vi "DataCollect.vi"() -> ()   [LabVIEW 2009]
uses:
  BaudRateSelector.ctl
  GlobalVariables.vi
  <vilib>/Platform/TimedLoop/XDataNode/XDataNode.xnode
  <vilib>/Platform/TimedLoop/XDataNode/loadlvalarms.vi
  <vilib>/Platform/TimedLoop/XDataNode/timing_clust.ctl
  <vilib>/Platform/TimedLoop/XDataNode/nitl_modes.ctl
  <vilib>/Platform/TimedLoop/XDataNode/wakeup.ctl
  <vilib>/Utility/file.llb/Write To Spreadsheet File (I64).vi
  <vilib>/Utility/file.llb/Write To Spreadsheet File (DBL).vi
  <vilib>/Utility/file.llb/Write To Spreadsheet File (string).vi
  <vilib>/Platform/TimedLoop/XDataNode/XDNodeRunTimeDep.lvlib
panel:
  in  "Reset Trial #":bool
  in  "Position Trial":bool
  in  "Trial #":i32=1 min=1 step=1
  in  "Experiment #":i32 min=0 step=1
  out "RH Cal Warning":bool
  in  "RH Calibration":string="RH_Calibration1.cal"
  out "LH Cal Warning":bool
  in  "LH Calibration":string="LH_Calibration1.cal"
  in  "Subject Initials":string="Default"
  in  "Start/Mark":bool
  out "RH Raw":u8[](array[numeric])
  out "RH Degrees":dbl[](array[numeric]) format="%7.2f"
  out "Sensor Names":string[](array[string])
  out "LH Degrees":dbl[](array[numeric]) format="%7.2f"
  out "LH Raw":u8[](array[numeric])
  out "RH Movement":dbl(graph)
  in  "RH Glove":bool=TRUE
  in  "LH Glove":bool=TRUE
  in  "Polhemus":bool=TRUE
  out "LH Movement":dbl(graph)
  out "Time":dbl
  out "Hand Position Graph":cluster{sgl, sgl}[](graph)
  in  "stop":bool
  in  "RH COM Port":refnum<visa-resource-name>="COM2"
  in  "LH COM Port":refnum<visa-resource-name>="COM1"
  out "Titles":string[](array[string])
  out "Interpreted Values":sgl[](array[numeric]) format="%.2f"
  in  "Parity":enum16{"None", "Odd", "Even", "Mark", "Space"}(ring)
  in  "Data Bits":u16=8 min=7 max=8 step=1
  in  "Baud Rate":T1=115200 items=["1200"=1200, "2400"=2400, "4800"=4800, "9600"=9600, "19200"=19200, "38400"=38400, "57600"=57600, "115200"=115200]
  in  "Polhemus COM Port":refnum<visa-resource-name>="COM3"
  # "(Pg Down)"
  # "(Pg Up)"
  # "Collect Data From:"
  # "If Data Bits = 8, Parity must be \"None\""
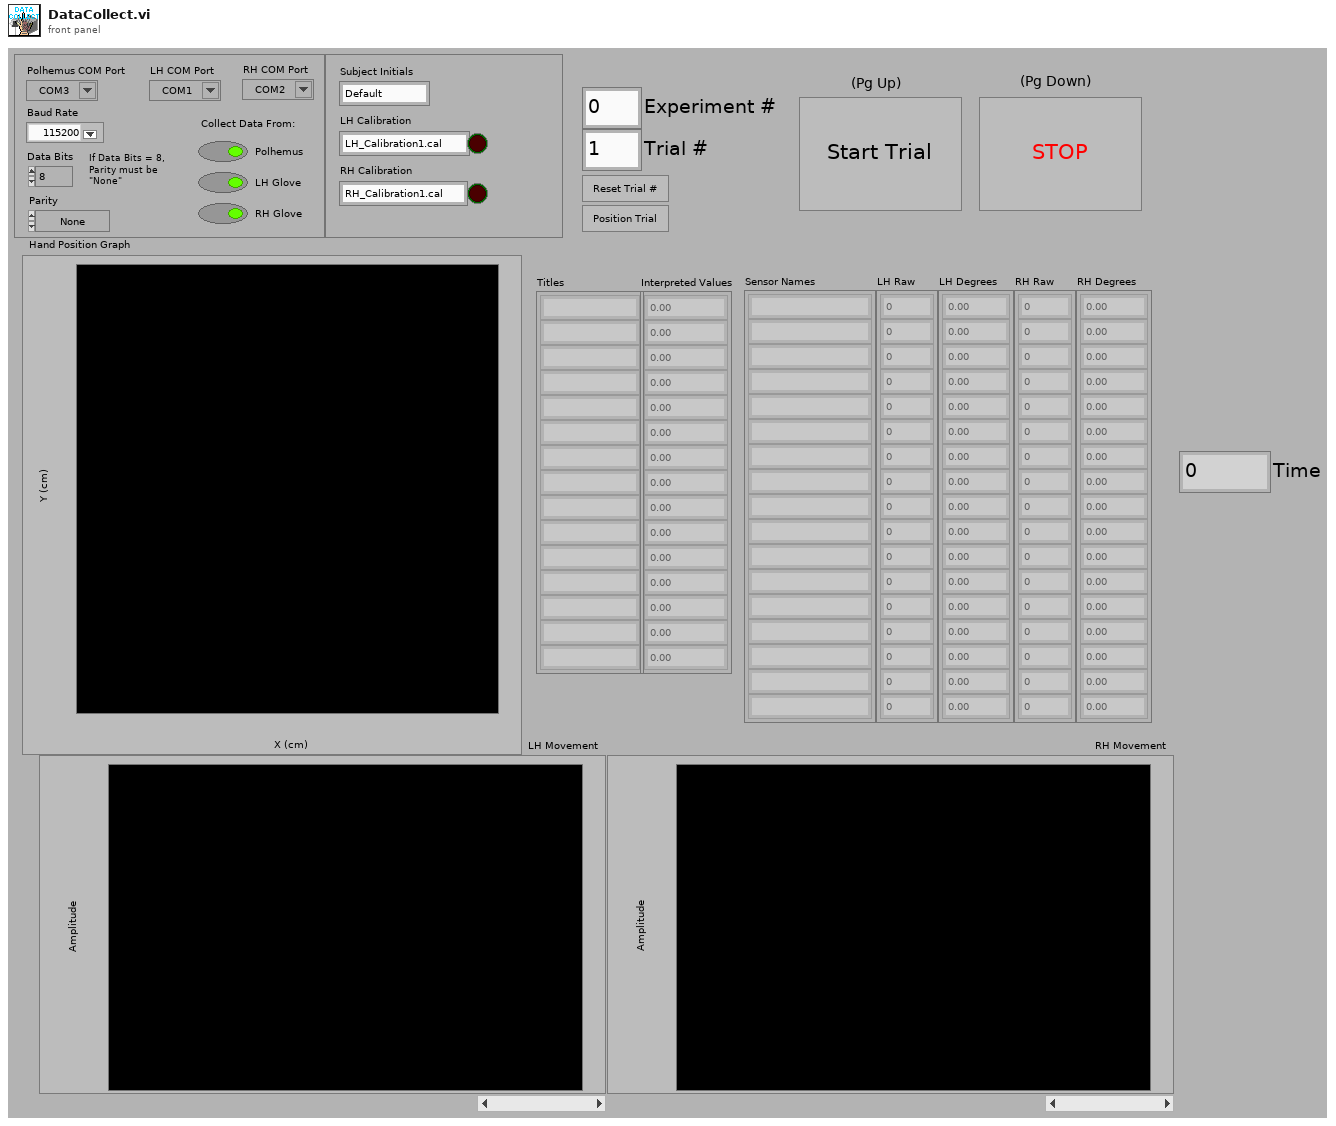
[diagram p1: front panel]
types:
  T1 = typedef "BaudRateSelector.ctl" = u32
  T2 = enum8{"Enabled", "Disabled", "Disabled and Grayed Out"}
  T3 = cluster{"#Bytes":i32[], "Titles":string[], "Format":enum16{"ASCII", "Binary"}, "Units":enum16{"Inches", "Centimeters"}, "Station State":bool[], "#Line Feeds":i32}
  T4 = typedef "XDNodeRunTimeDep.lvlib/timing_clust.ctl" = cluster{"Expected End [f-1]":u64, "Actual End [f-1]":u64, "Finished Late? [f-1]":bool, "Expected End [i-1]":u64, "Actual End [i-1]":u64, "Finished Late? [i-1]":bool, "Expected Start [i]":u64, "Actual Start [i]":u64, "Expected Start [f]":u64, "Actual Start [f]":u64, "Source Name":string, "Structure Name":string, "Period":i64, "Deadline":i64, "Offset":i64, "Start":i64, "Priority":i32, "Timeout":i32, "Mode":T5, "Wakeup Reason":T6, "Error":errorcluster, "Source Type":string, "Secondary Source Type":string, "Global End Time":u64, "Global Start Time":u64, "Frame Duration":u64, "Iteration Duration":u64, "Assigned CPU":i32, "I/O Scan Engine Mode":u32}
  T5 = typedef "XDNodeRunTimeDep.lvlib/nitl_modes.ctl" = enum32{"No Change", "Process missed periods, maintain original phase", "Discard missed periods, maintain original phase", "Process missed periods, ignore original phase", "Discard missed periods, ignore original phase"}
  T6 = typedef "XDNodeRunTimeDep.lvlib/wakeup.ctl" = enum32{"Normal", "Aborted", "Asynchronous wakeup", "Timing source error", "Timed loop error", "Timeout"}
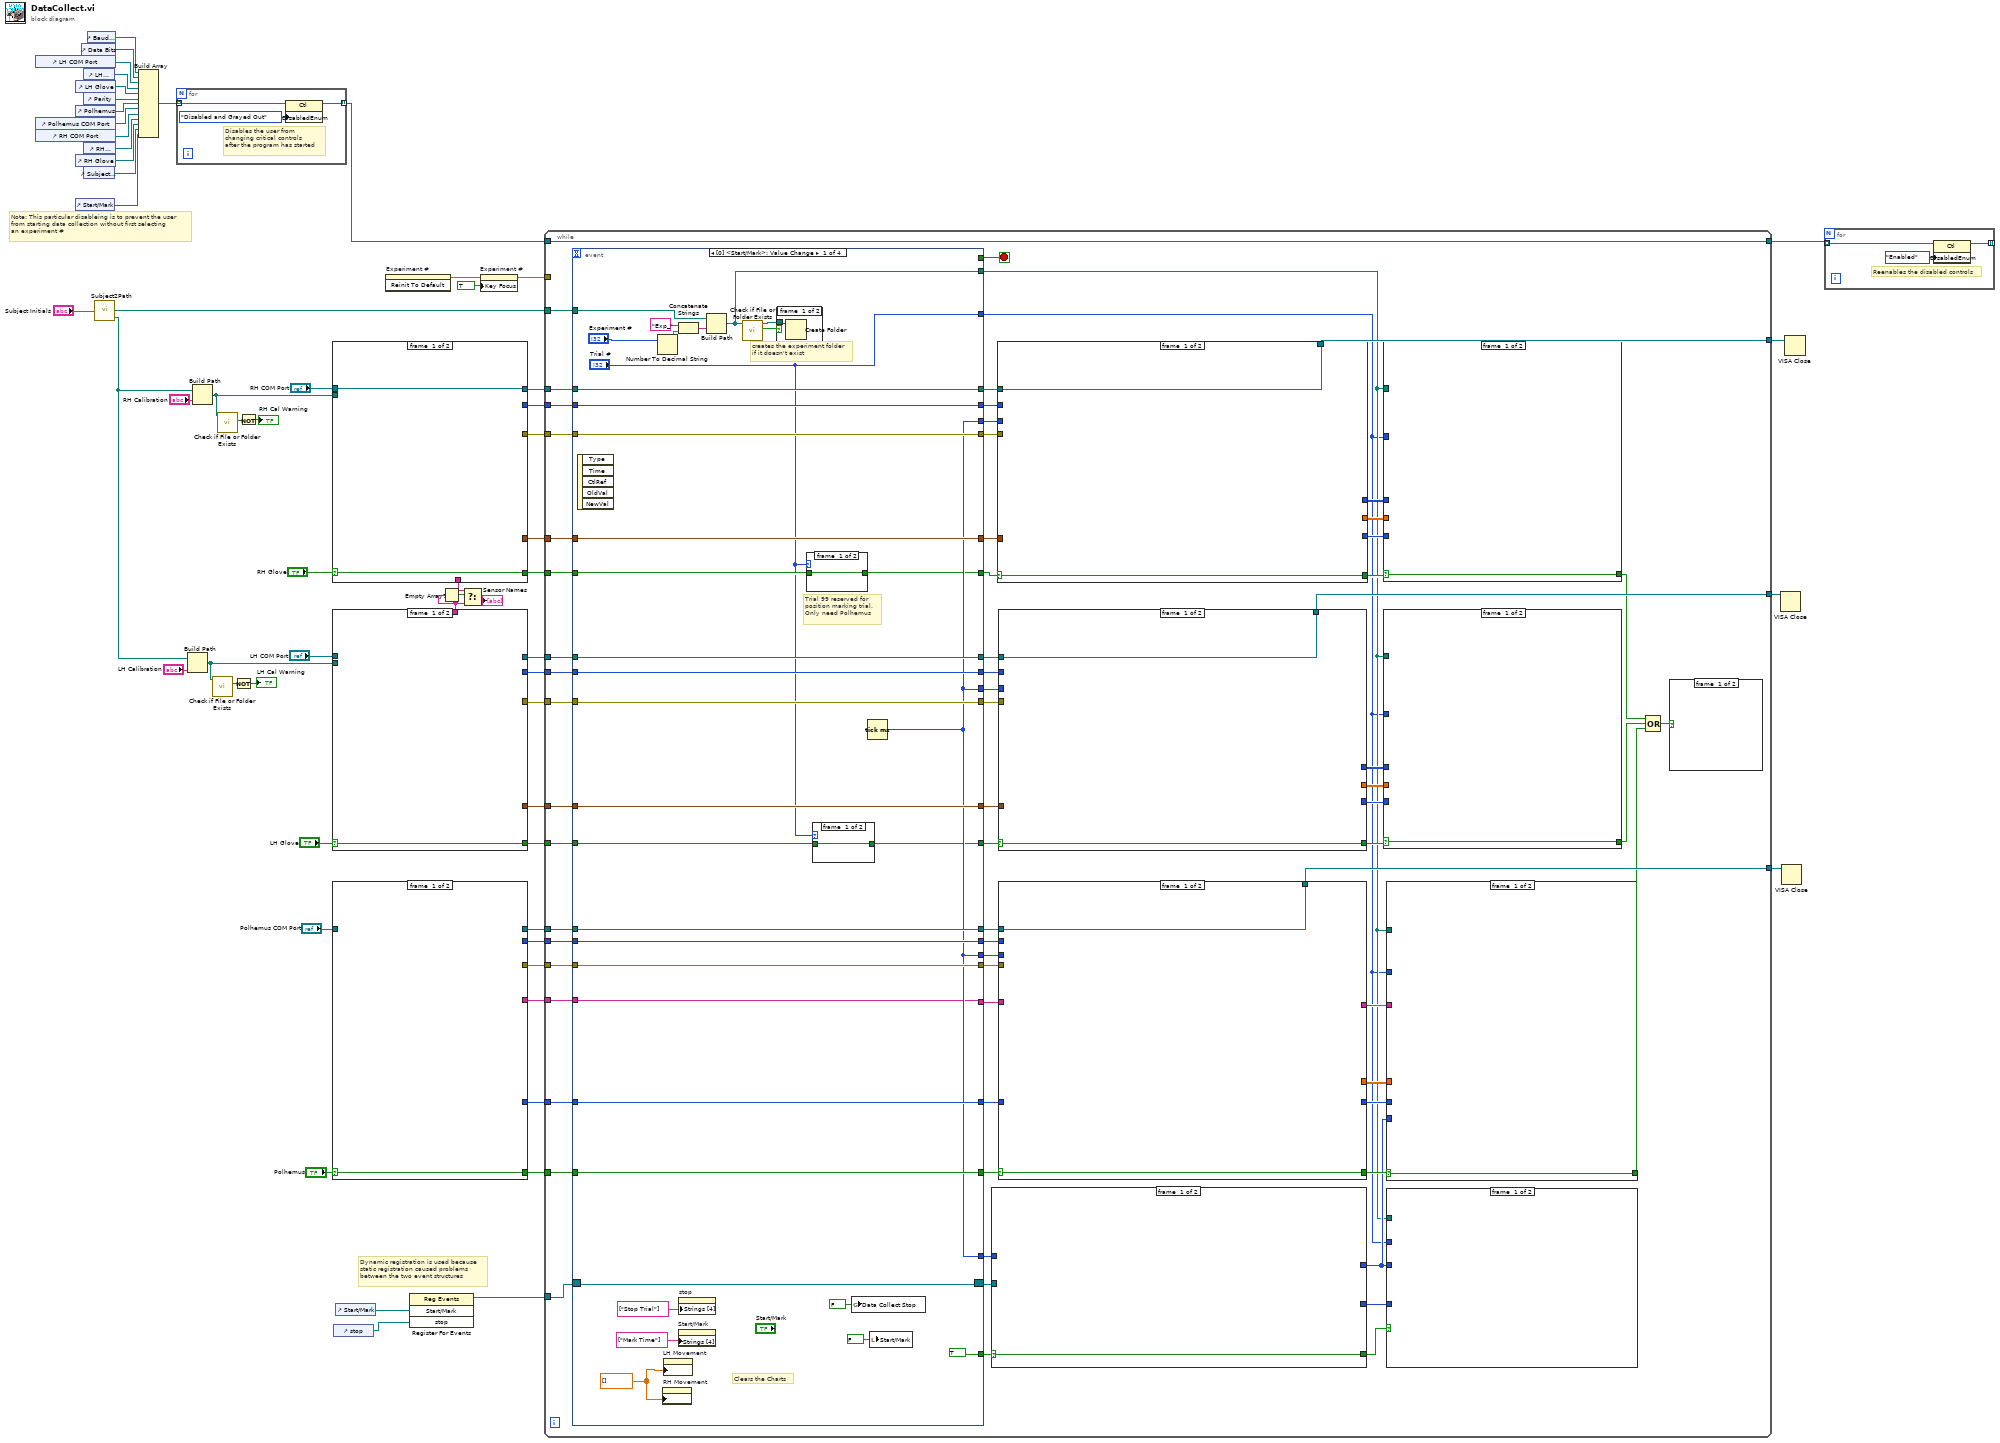
[diagram p0: block diagram]
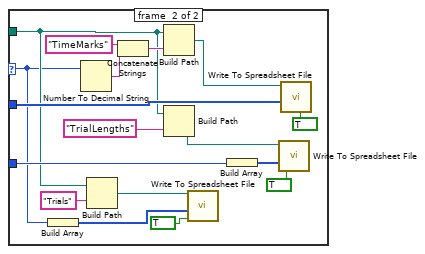
[diagram p3: hidden frame]
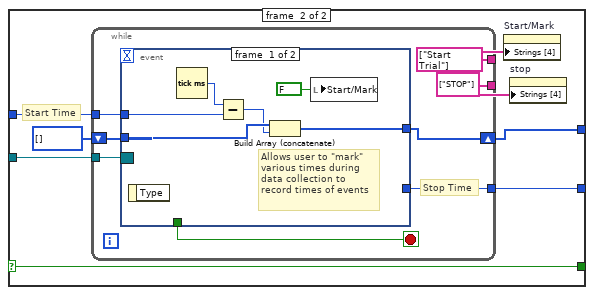
[diagram p4: hidden frame]
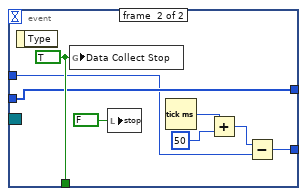
[diagram p5: hidden frame]
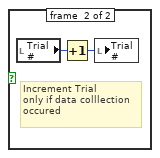
[diagram p6: hidden frame]
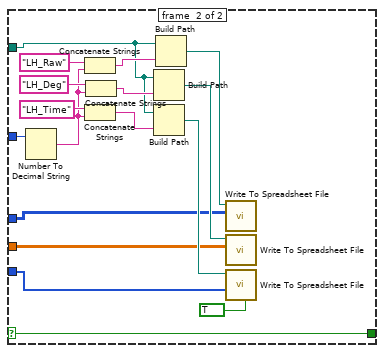
[diagram p7: hidden frame]
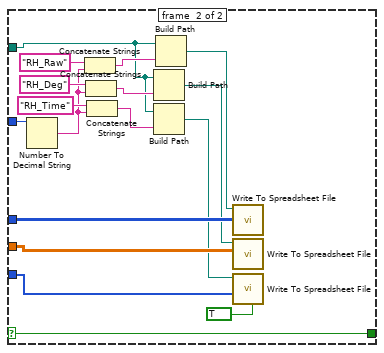
[diagram p8: hidden frame]
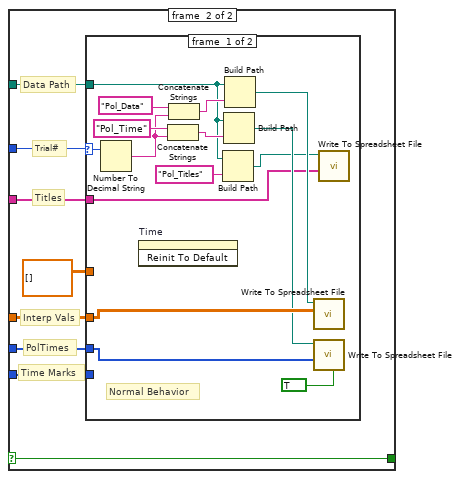
[diagram p9: hidden frame]
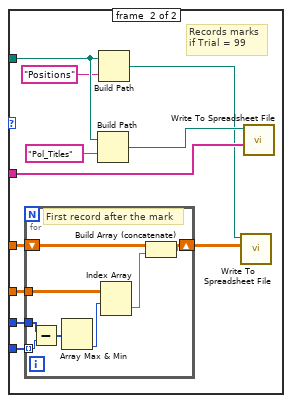
[diagram p10: hidden frame]
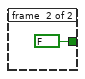
[diagram p11: hidden frame]
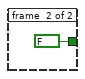
[diagram p12: hidden frame]
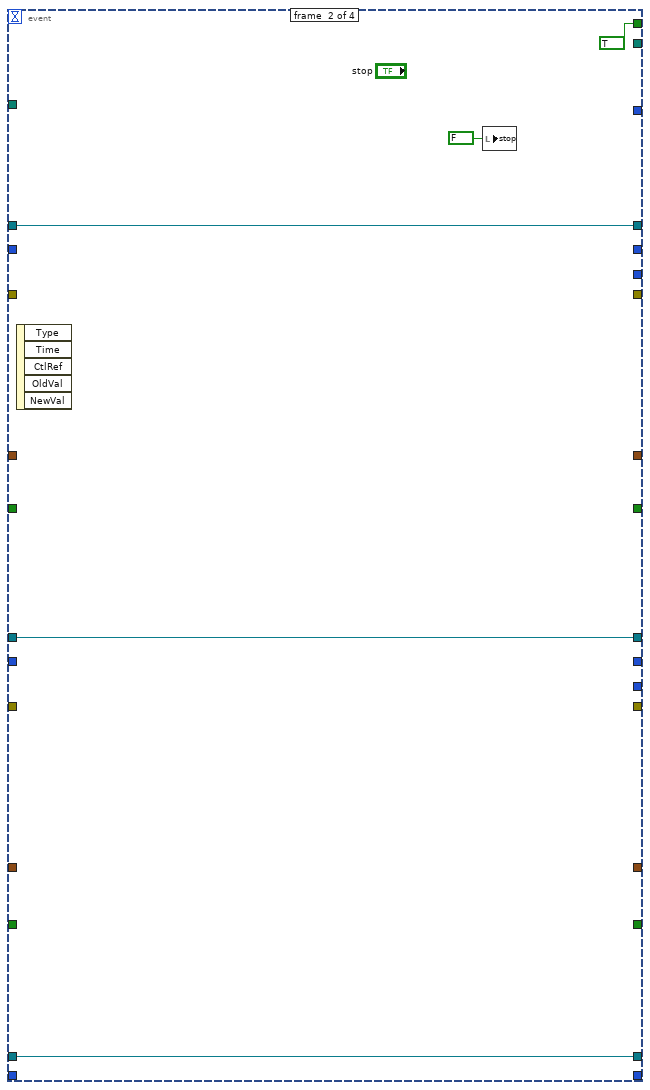
[diagram p14: hidden frame]
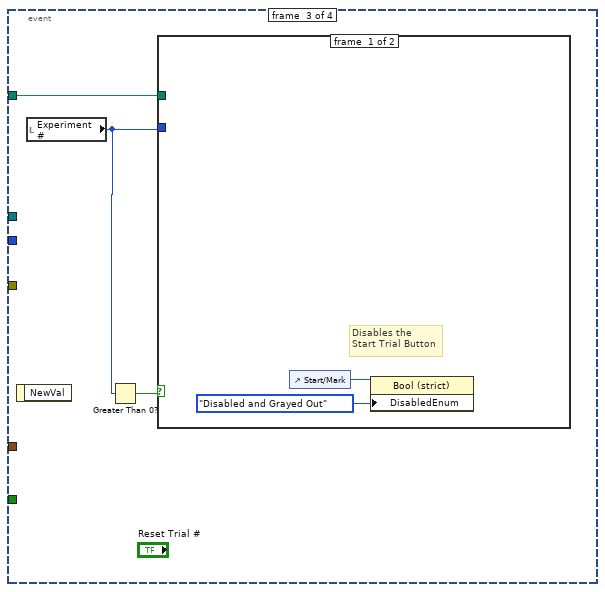
[diagram p15: hidden frame]
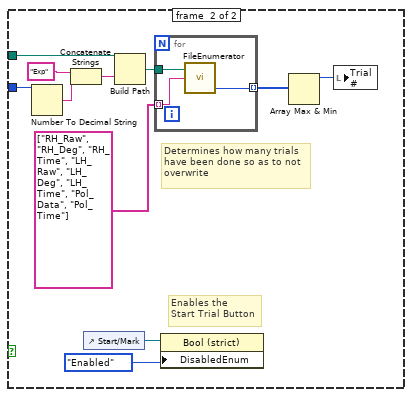
[diagram p16: hidden frame]
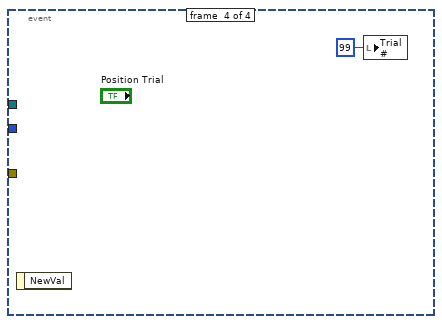
[diagram p17: hidden frame]
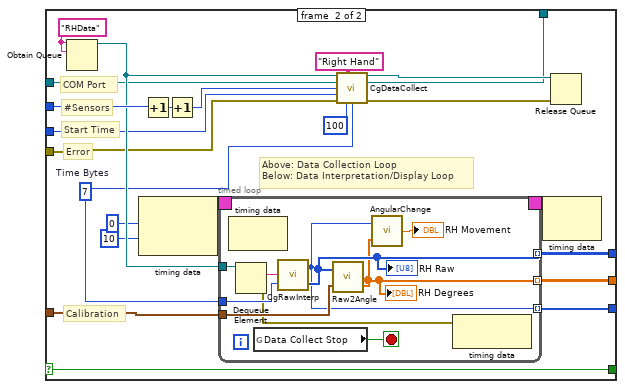
[diagram p18: hidden frame]
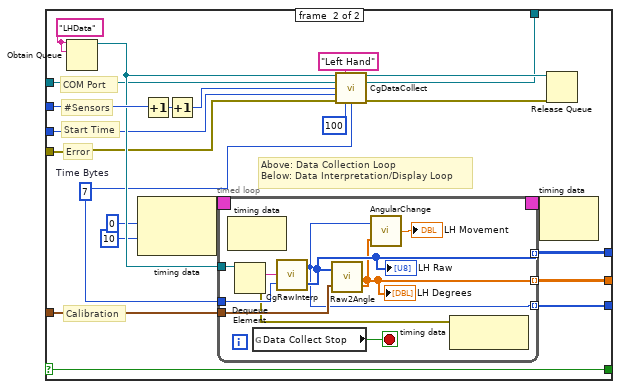
[diagram p19: hidden frame]
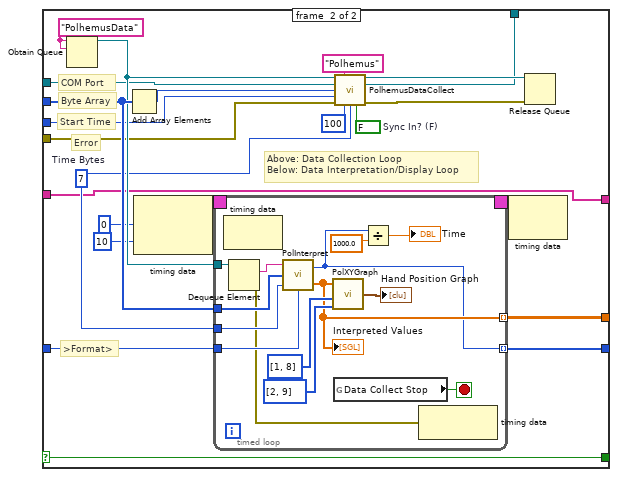
[diagram p20: hidden frame]
diagram:
  # "Dynamic registration is used because\nstatic registration caused problems\nbetween the two event structures"
  # "Note: This particular disableing is to prevent the user\nfrom starting data collection without first selecting\nan experiment #"
  n1 = control-ref of="LH COM Port"() -> (w36:refnum<vi>)
  n2 = control-ref of="Polhemus COM Port"() -> (w31:refnum<vi>)
  n3 = control-ref of="RH COM Port"() -> (w30:refnum<vi>)
  n4 = control-ref of="Start/Mark"() -> (w11:refnum<vi>)
  n5 = control-ref of="LH Glove"() -> (w34:refnum<vi>)
  n6 = control-ref of="Polhemus"() -> (w32:refnum<vi>)
  n7 = control-ref of="RH Glove"() -> (w28:refnum<vi>)
  n8 = control-ref of="Data Bits"() -> (w37:refnum<vi>)
  n9 = control-ref of="LH Calibration"() -> (w35:refnum<vi>)
  n10 = control-ref of="Subject Initials"() -> (w27:refnum<vi>)
  n11 = control-ref of="Parity"() -> (w33:refnum<vi>)
  n12 = control-ref of="RH Calibration"() -> (w29:refnum<vi>)
  n13 = control-ref of="Baud Rate"() -> (w26:refnum<vi>)
  n14 = call "Subject2Path.vi"("Subject Initials"="Subject Initials") -> ("Data Path"=w23:path, "Calibration Path"=w14:path)  [unwired: 1 in, 1 out]
  n15 = Build Array(w26, w37, w36, w35, w34, w33, w32, w31, w30, w29, w28, w27, w11) -> (w25:refnum<vi>[])
  n16 = for {
    tunnel: w25 -> [w65] mode=indexing
    tunnel: [w63] -> w13 mode=indexing
    # "Disables the user from\nchanging critical controls\nafter the program has started"
    n17 = property class="Ctl"(reference=w65, "DisabledEnum"=T2."Disabled and Grayed Out" ("Disabled")) -> (reference out=w63:refnum<vi>)  [unwired: 1 in, 1 out]
  }
  n18 = Build Path(base path=w14, name or relative path="LH Calibration") -> (appended path=w17:path)
  n19 = Build Path(base path=w14, name or relative path="RH Calibration") -> (appended path=w21:path)
  n20 = call <vilib>:"Check if File or Folder Exists.vi"("path"=w17) -> ("file or folder exists?"=w16:bool)  [unwired: 8 in, 2 out]
  n21 = call <vilib>:"Check if File or Folder Exists.vi"("path"=w21) -> ("file or folder exists?"=w20:bool)  [unwired: 8 in, 2 out]
  n22 = Not(x=w16) -> (.not. x?=→"LH Cal Warning":bool)
  n23 = Not(x=w20) -> (.not. x?=→"RH Cal Warning":bool)
  n24 = case shown="True" "RH Glove" {
    selector: "RH Glove" -> [w67 w69]
    tunnel: [w66 w75] -> w47
    tunnel: [_ w74] -> w46
    tunnel: [_ w73] -> w45
    tunnel: [_ w72] -> w44
    tunnel: [_ w71] -> w56
    tunnel: [w67 w69] -> w43
    tunnel: "RH COM Port" -> [w66 w70]
    tunnel: w21 -> [_ w68]
    frame #0 {
    }
    frame #1 {
      # "Initializes the RH Glove"
      n25 = call "CgInit.vi"("Calibration File"=w68, "VISA resource name"=w70) -> ("error out"=w73:errorcluster, "Sensor Names"=w71:string[], "#Sensors"=w74:i32, "VISA resource name out"=w75:refnum<visa-resource-name>, "Calibration Array"=w72:cluster{"Offset":dbl, "Gain":dbl}[])  [unwired: 3 in]
    }
  }
  n26 = case shown="True" "LH Glove" {
    selector: "LH Glove" -> [w76 w78]
    tunnel: [_ w84] -> w62
    tunnel: [_ w83] -> w41
    tunnel: [_ w82] -> w61
    tunnel: [_ w81] -> w40
    tunnel: [_ w80] -> w53
    tunnel: [w76 w78] -> w51
    tunnel: "LH COM Port" -> [_ w79]
    tunnel: w17 -> [_ w77]
    frame #0 {
    }
    frame #1 {
      # "Initializes the LH Glove"
      n27 = call "CgInit.vi"("Calibration File"=w77, "VISA resource name"=w79) -> ("error out"=w81:errorcluster, "Sensor Names"=w80:string[], "#Sensors"=w84:i32, "VISA resource name out"=w83:refnum<visa-resource-name>, "Calibration Array"=w82:cluster{"Offset":dbl, "Gain":dbl}[])  [unwired: 3 in]
    }
  }
  n28 = case shown="True" "Polhemus" {
    selector: "Polhemus" -> [w85 w88]
    tunnel: [_ w96] -> w60
    tunnel: [_ w95] -> w59
    tunnel: [_ w94] -> w58
    tunnel: [_ w93] -> w57
    tunnel: [w85 w88] -> w52
    tunnel: "Polhemus COM Port" -> [_ w87]
    tunnel: [_ w86] -> w7
    frame #0 {
    }
    frame #1 {
      # "Initializes the Polhemus"
      n29 = call "PolInit.vi"("VISA resource name"=w87, "Baud Rate"="Baud Rate", "Data Bits"="Data Bits", "Parity"="Parity") -> ("VISA resource name out"=w94:refnum<visa-resource-name>, "Polhemus Info"=w89:T3, "error out"=w93:errorcluster)  [unwired: 9 in]
      n30 = Unbundle By Name(w89) -> ("#Bytes"=w96:i32[], "Titles"=w86:string[], "Format"=w95:enum16{"ASCII", "Binary"})  [unwired: 2 out]
      "Titles" <- w86
    }
  }
  n31 = control-ref of="stop"() -> (w4:refnum<vi>)
  n32 = control-ref of="Start/Mark"() -> (w6:refnum<vi>)
  n33 = invoke on="Experiment #" class="DigNum (strict)" method="Reinit To Default"() -> (error out=w3:errorcluster)  [unwired: 3 in, 2 out]
  n34 = register-events(w6, w4) -> (reference out=w5:refnum<event-registration>)  [unwired: 2 in, 1 out]
  n35 = Empty Array?(array=w53) -> (empty?=w55:bool)
  n36 = Select(t=w56, s=w55, f=w53) -> (s? t:f=→"Sensor Names":string[])
  n37 = property on="Experiment #" class="DigNum (strict)"(error in=w3, "Key Focus"=TRUE) -> (error out=w2:errorcluster)  [unwired: 1 in, 1 out]
  n38 = while {
    tunnel: w62 -> [w156]
    tunnel: w61 -> [w154]
    tunnel: w60 -> [w151]
    tunnel: w59 -> [w149]
    tunnel: w58 -> [w152]
    tunnel: w57 -> [w150]
    tunnel: w52 -> [w148]
    tunnel: w51 -> [w153]
    tunnel: w47 -> [w162]
    tunnel: w46 -> [w161]
    tunnel: w45 -> [w160]
    tunnel: w44 -> [w159]
    tunnel: w43 -> [w158]
    tunnel: w41 -> [w157]
    tunnel: w40 -> [w155]
    tunnel: w23 -> [w128]
    tunnel: w13 -> [w127]
    tunnel: [w127] -> w12
    tunnel: [w126] -> w8
    tunnel: [w125] -> w9
    tunnel: [w124] -> w10
    tunnel: w7 -> [w108]
    tunnel: w5 -> [w103]
    tunnel: w2 -> [_]
    stop <- w129 stop-if-true
    n39 = event shown="[0] <Start/Mark>: Value Change" {
      selector: w103 -> [w303 _ _ _]
      dyn-events: [w303 _ _ _] -> w102
      timeout: _ -> [_ _ _ _]
      tunnel: w162 -> [w321 w340 _ _]
      tunnel: w161 -> [w322 _ _ _]
      tunnel: w160 -> [w323 _ _ _]
      tunnel: w159 -> [w324 _ _ _]
      tunnel: w158 -> [w300 _ _ _]
      tunnel: w157 -> [w312 w339 _ _]
      tunnel: w156 -> [w311 _ _ _]
      tunnel: w155 -> [w310 _ _ _]
      tunnel: w154 -> [w325 _ _ _]
      tunnel: w153 -> [w298 _ _ _]
      tunnel: w152 -> [w326 w338 _ _]
      tunnel: w151 -> [w327 _ _ _]
      tunnel: w150 -> [w328 _ _ _]
      tunnel: w149 -> [w329 _ _ _]
      tunnel: w148 -> [w330 _ _ _]
      tunnel: [w330 _ _ _] -> w147
      tunnel: [w329 _ _ _] -> w146
      tunnel: [w328 _ _ _] -> w145
      tunnel: [w327 _ _ _] -> w144
      tunnel: [w326 w338 _ _] -> w143
      tunnel: [w297 _ _ _] -> w142
      tunnel: [w325 _ _ _] -> w141
      tunnel: [w310 _ _ _] -> w140
      tunnel: [w311 _ _ _] -> w139
      tunnel: [w312 w339 _ _] -> w138
      tunnel: [w299 _ _ _] -> w137
      tunnel: [w324 _ _ _] -> w136
      tunnel: [w323 _ _ _] -> w135
      tunnel: [w322 _ _ _] -> w134
      tunnel: [w321 w340 _ _] -> w133
      tunnel: [w309 _ _ _] -> w105
      tunnel: [w309 _ _ _] -> w132
      tunnel: [w309 _ _ _] -> w131
      tunnel: [w309 _ _ _] -> w130
      tunnel: [_ TRUE ("stop") _ _] -> w129
      tunnel: w128 -> [w318 _ w342 _]
      tunnel: [w315 _ _ _] -> w99
      tunnel: ["Trial #" _ _ _] -> w98
      tunnel: [w306 _ _ _] -> w107
      tunnel: w108 -> [w306 _ _ _]
      tunnel: [TRUE _ _ _] -> w101
      event #0 {
        w308 = dbl[] [] ("History Data")
        # "Trial 99 reserved for\nposition marking trial.\nOnly need Polhemus"
        # "Clears the Charts"
        # "creates the experiment folder\nif it doesn't exist"
        n40 = event-data() -> ()  [unwired: 1 in, 5 out]
        n41 = Number To Decimal String(number="Experiment #") -> (decimal integer string=w319:string)  [unwired: 1 in]
        n42 = property on="RH Movement" class="WFChart (strict)"("History Data"=w308) -> ()  [unwired: 2 in, 2 out]
        n43 = property on="LH Movement" class="WFChart (strict)"("History Data"=w308) -> ()  [unwired: 2 in, 2 out]
        n44 = Concatenate Strings("Exp_", w319) -> (w317:string)
        n45 = property on="Start/Mark" class="Bool (strict)"("Strings [4]"=string[] ["Mark Time"]) -> ()  [unwired: 2 in, 2 out]
        n46 = property on="stop" class="Bool (strict)"("Strings [4]"=string[] ["Stop Trial"]) -> ()  [unwired: 2 in, 2 out]
        n47 = Build Path(base path=w318, name or relative path=w317) -> (appended path=w315:path)
        n48 = call <vilib>:"Check if File or Folder Exists.vi"("path"=w315) -> ("file or folder exists?"=w314:bool, "dup path"=w313:path)  [unwired: 8 in, 1 out]
        n49 = case shown="False" w314 {
          tunnel: w313 -> [w335 _]
          frame #0 {
            n50 = Create Folder(path (use dialog)=w335) -> ()  [unwired: 2 in, 3 out]
          }
          frame #1 {
          }
        }
        n51 = case shown="Default" "Trial #" {
          tunnel: w300 -> [w333 _]
          tunnel: [w333 FALSE] -> w299
          frame #0 {
          }
          frame #1 {
          }
        }
        n52 = case shown="Default" "Trial #" {
          tunnel: w298 -> [w331 _]
          tunnel: [w331 FALSE] -> w297
          frame #0 {
          }
          frame #1 {
          }
        }
        n53 = global write "GlobalVariables.vi" "Data Collect Stop"(FALSE ("Data Collect Stop")) -> ()
        n54 = Tick Count (ms)() -> (millisecond timer value=w309:u32)
        n55 = local write "Start/Mark"(FALSE ("Start/Mark")) -> ()
      }
      event #1 {
        n56 = event-data() -> ()  [unwired: 1 in, 5 out]
        n57 = local write "stop"(FALSE ("stop")) -> ()
      }
      event #2 {
        n58 = event-data() -> ()  [unwired: 1 in, 1 out]
        n59 = local read "Experiment #"() -> (w341:i32)
        n60 = Greater Than 0?(x=w341) -> (x > 0?=w343:bool)
        n61 = case shown="True" w343 {
          tunnel: w342 -> [_ w351]
          tunnel: w341 -> [_ w354]
          frame #0 {
            # "Disables the\nStart Trial Button"
            n62 = control-ref of="Start/Mark"() -> (w344:refnum<vi>)
            n63 = property class="Bool (strict)"(reference=w344, "DisabledEnum"=T2."Disabled and Grayed Out" ("Disabled")) -> ()  [unwired: 1 in, 2 out]
          }
          frame #1 {
            # "Determines how many trials have been done so as to not overwrite"
            # "Enables the\nStart Trial Button"
            n64 = Number To Decimal String(number=w354) -> (decimal integer string=w352:string)  [unwired: 1 in]
            n65 = Concatenate Strings("Exp", w352) -> (w350:string)
            n66 = control-ref of="Start/Mark"() -> (w356:refnum<vi>)
            n67 = Build Path(base path=w351, name or relative path=w350) -> (appended path=w349:path)
            n68 = for {
              tunnel: w349 -> [w358]
              tunnel: string[] ["RH_Raw", "RH_Deg", "RH_Time", "LH_Raw", "LH_Deg", "LH_Time", "Pol_Data", "Pol_Time"] -> [w359] mode=indexing
              tunnel: [w357] -> w347 mode=indexing
              n69 = call "FileEnumerator.vi"("Filename"=w359, "Path"=w358) -> ("Number"=w357:i32)  [unwired: 1 in, 2 out]
            }
            n70 = property class="Bool (strict)"(reference=w356, "DisabledEnum"=T2."Enabled" ("Disabled")) -> ()  [unwired: 1 in, 2 out]
            n71 = Array Max & Min(array=w347) -> (max value=w346:i32)  [unwired: 3 out]
            n72 = local write "Trial #"(w346) -> ()
          }
        }
      }
      event #3 {
        n73 = event-data() -> ()  [unwired: 1 in, 1 out]
        n74 = local write "Trial #"(99 ("Trial #")) -> ()
      }
    }
    n75 = case shown="True" w101 {
      selector: w101 -> [w184 w191]
      tunnel: w105 -> [_ w192]
      tunnel: [w184 w191] -> w104
      tunnel: [_ w190] -> w100
      tunnel: w102 -> [_ w187]
      tunnel: [_ w185] -> w97
      frame #0 {
      }
      frame #1 {
        # "Start Time"
        n76 = while {
          tunnel: w192 -> [w200]
          shift-right: [w199] -> w190
          shift-left: u32[] [] -> [w198]
          tunnel: [string[] ["Start Trial"] ("Strings [4]")] -> w189
          tunnel: [string[] ["STOP"] ("Strings [4]")] -> w188
          tunnel: w187 -> [w194]
          tunnel: [w193] -> w185
          stop <- w197 stop-if-true
          # "Stop Time"
          n77 = event shown="[1] <stop>: Value Change" {
            selector: w194 -> [_ _]
            dyn-events: _ -> [_ _]
            timeout: _ -> [_ _]
            tunnel: w200 -> [w205 w211]
            tunnel: [w204 w213] -> w199
            tunnel: w198 -> [w203 w213]
            tunnel: [_ w214] -> w197
            tunnel: [_ w210] -> w193
            event #0 {
              # "Allows user to \"mark\"\nvarious times during\ndata collection to\nrecord times of events"
              n78 = event-data() -> ()  [unwired: 1 in, 1 out]
              n79 = Tick Count (ms)() -> (millisecond timer value=w206:u32)
              n80 = Subtract(x=w206, y=w205) -> (x-y=w201:u32)
              n81 = Build Array (concatenate)(w203, w201) -> (w204:u32[])
              n82 = local write "Start/Mark"(FALSE ("Start/Mark")) -> ()
            }
            event #1 {
              w214 = TRUE ("Data Collect Stop")
              n83 = event-data() -> ()  [unwired: 1 in, 1 out]
              n84 = global write "GlobalVariables.vi" "Data Collect Stop"(w214) -> ()
              n85 = local write "stop"(FALSE ("stop")) -> ()
              n86 = Tick Count (ms)() -> (millisecond timer value=w209:u32)
              n87 = Add(x=w209, y=u32 50) -> (x+y=w207:u32)
              n88 = Subtract(x=w207, y=w211) -> (x-y=w210:u32)
            }
          }
        }
        n89 = property on="Start/Mark" class="Bool (strict)"("Strings [4]"=w189) -> ()  [unwired: 2 in, 2 out]
        n90 = property on="stop" class="Bool (strict)"("Strings [4]"=w188) -> ()  [unwired: 2 in, 2 out]
      }
    }
    n91 = case shown="True" w137 {
      selector: w137 -> [w361 w364]
      tunnel: w134 -> [_ w383]
      tunnel: w136 -> [_ w381]
      tunnel: w133 -> [w362 w378]
      tunnel: w130 -> [_ w372]
      tunnel: w135 -> [_ w371]
      tunnel: [_ w370] -> w122
      tunnel: [_ w369] -> w121
      tunnel: [w362 w365] -> w124
      tunnel: [w361 w364] -> w123
      tunnel: [_ w363] -> w109
      frame #0 {
      }
      frame #1 {
        w366 = i16 7  # Time Bytes
        w376 = "RHData" ("name (unnamed)")
        # "Above: Data Collection Loop\nBelow: Data Interpretation/Display Loop"
        # "Calibration"
        # "Error"
        # "Start Time"
        # "#Sensors"
        # "COM Port"
        n92 = Obtain Queue(name (unnamed)=w376, element data type=w376) -> (queue out=w379:refnum<queue>)  [unwired: 3 in, 2 out]
        n93 = node-c288(i64 0 ("Period"), 10 ("Priority")) -> (w385:T4)
        n94 = Increment(x=w383) -> (x+1=w382:i32)
        n95 = Increment(x=w382) -> (x+1=w377:i32)
        n96 = timed-loop {
          tunnel: w379 -> [w395]
          tunnel: w381 -> [w394]
          timing: w385 -> [_]
          timing-out: [_] -> w384
          tunnel: [w393] -> w370 mode=indexing
          tunnel: [w388] -> w369 mode=indexing
          tunnel: w366 -> [w391]
          tunnel: [w386] -> w363 mode=indexing
          stop <- w389 stop-if-true
          n97 = node-c288() -> ()  [unwired: 1 in, 1 out]
          n98 = Dequeue Element(queue=w395) -> (element=w392:string, error out=w387:errorcluster)  [unwired: 2 in, 2 out]
          n99 = global read "GlobalVariables.vi" "Data Collect Stop"() -> (w389:bool)
          n100 = call "CgRawInterp.vi"("Time Bytes Before Output"=w391, "Cyberglove Out"=w392) -> ("Raw Data"=w393:u8[], "Time"=w386:i32)
          "RH Raw" <- w393
          n101 = call "Raw2Angle.vi"("Calibration"=w394, "Raw Data"=w393) -> ("Degrees"=w388:dbl[])  [unwired: 1 out]
          "RH Degrees" <- w388
          n102 = call "AngularChange.vi"("Degrees"=w388, "Time"=w386) -> ("Angular Change"=→"RH Movement":dbl)
          n103 = node-c288(w387) -> ()  [unwired: 1 out]
        }
        n104 = call "CgDataCollect.vi"("Data Queue"=w379, "Timed Structure Name"="Right Hand", "VISA resource name"=w378, "Bytes to Read"=w377, "Relative Time"=w372, "error in (no error)"=w371, "Time Loop Priority"=100, "Time Bytes Before Output"=w366) -> ("Queue Out"=w374:refnum<queue>, "VISA resource name out"=w365:refnum<visa-resource-name>, "error out"=w373:errorcluster)  [unwired: 4 in, 1 out]
        n105 = node-c288(w384) -> ()  [unwired: 1 out]
        n106 = Release Queue(queue=w374, error in (no error)=w373) -> ()  [unwired: 1 in, 3 out]
      }
    }
    n107 = case shown="True" w142 {
      selector: w142 -> [w405 w408]
      tunnel: w139 -> [_ w427]
      tunnel: w141 -> [_ w425]
      tunnel: w138 -> [w406 w422]
      tunnel: w131 -> [_ w416]
      tunnel: w140 -> [_ w415]
      tunnel: [_ w414] -> w120
      tunnel: [_ w413] -> w119
      tunnel: [w406 w409] -> w125
      tunnel: [w405 w408] -> w118
      tunnel: [_ w407] -> w111
      frame #0 {
      }
      frame #1 {
        w410 = i16 7  # Time Bytes
        w420 = "LHData" ("name (unnamed)")
        # "Above: Data Collection Loop\nBelow: Data Interpretation/Display Loop"
        # "Calibration"
        # "Error"
        # "Start Time"
        # "#Sensors"
        # "COM Port"
        n108 = Obtain Queue(name (unnamed)=w420, element data type=w420) -> (queue out=w423:refnum<queue>)  [unwired: 3 in, 2 out]
        n109 = node-c288(i64 0 ("Period"), 10 ("Priority")) -> (w429:T4)
        n110 = Increment(x=w427) -> (x+1=w426:i32)
        n111 = Increment(x=w426) -> (x+1=w421:i32)
        n112 = timed-loop {
          tunnel: w423 -> [w439]
          tunnel: w425 -> [w438]
          timing: w429 -> [_]
          timing-out: [_] -> w428
          tunnel: [w437] -> w414 mode=indexing
          tunnel: [w432] -> w413 mode=indexing
          tunnel: w410 -> [w435]
          tunnel: [w430] -> w407 mode=indexing
          stop <- w433 stop-if-true
          n113 = node-c288() -> ()  [unwired: 1 in, 1 out]
          n114 = Dequeue Element(queue=w439) -> (element=w436:string, error out=w431:errorcluster)  [unwired: 2 in, 2 out]
          n115 = global read "GlobalVariables.vi" "Data Collect Stop"() -> (w433:bool)
          n116 = call "CgRawInterp.vi"("Time Bytes Before Output"=w435, "Cyberglove Out"=w436) -> ("Raw Data"=w437:u8[], "Time"=w430:i32)
          "LH Raw" <- w437
          n117 = call "Raw2Angle.vi"("Calibration"=w438, "Raw Data"=w437) -> ("Degrees"=w432:dbl[])  [unwired: 1 out]
          "LH Degrees" <- w432
          n118 = call "AngularChange.vi"("Degrees"=w432, "Time"=w430) -> ("Angular Change"=→"LH Movement":dbl)
          n119 = node-c288(w431) -> ()  [unwired: 1 out]
        }
        n120 = call "CgDataCollect.vi"("Data Queue"=w423, "Timed Structure Name"="Left Hand", "VISA resource name"=w422, "Bytes to Read"=w421, "Relative Time"=w416, "error in (no error)"=w415, "Time Loop Priority"=100, "Time Bytes Before Output"=w410) -> ("Queue Out"=w418:refnum<queue>, "VISA resource name out"=w409:refnum<visa-resource-name>, "error out"=w417:errorcluster)  [unwired: 4 in, 1 out]
        n121 = node-c288(w428) -> ()  [unwired: 1 out]
        n122 = Release Queue(queue=w418, error in (no error)=w417) -> ()  [unwired: 1 in, 3 out]
      }
    }
    n123 = case shown="True" w147 {
      selector: w147 -> [w449 w453]
      tunnel: w144 -> [_ w471]
      tunnel: w146 -> [_ w470]
      tunnel: [_ w469] -> w116
      tunnel: w143 -> [w450 w466]
      tunnel: w145 -> [_ w465]
      tunnel: w132 -> [_ w459]
      tunnel: [w450 w454] -> w126
      tunnel: [w449 w453] -> w117
      tunnel: [_ w452] -> w110
      tunnel: [_ w451] -> w106
      tunnel: w107 -> [_ w451]
      frame #0 {
      }
      frame #1 {
        w455 = 7  # Time Bytes
        w458 = FALSE  # Sync In? (F)
        w460 = "PolhemusData" ("name (unnamed)")
        # "Above: Data Collection Loop\nBelow: Data Interpretation/Display Loop"
        # ">Format>"
        # "Error"
        # "Start Time"
        # "Byte Array"
        # "COM Port"
        n124 = Obtain Queue(name (unnamed)=w460, element data type=w460) -> (queue out=w467:refnum<queue>)  [unwired: 3 in, 2 out]
        n125 = Add Array Elements(numeric array=w471) -> (sum=w464:i32)
        n126 = node-c288(i64 0 ("Period"), 10 ("Priority")) -> (w473:T4)
        n127 = timed-loop {
          tunnel: w467 -> [w487]
          tunnel: w471 -> [w485]
          tunnel: w470 -> [w484]
          tunnel: [w480] -> w469 mode=indexing
          timing: w473 -> [_]
          timing-out: [_] -> w472
          tunnel: w455 -> [w479]
          tunnel: [w475] -> w452 mode=indexing
          stop <- w478 stop-if-true
          n128 = node-c288() -> ()  [unwired: 1 in, 1 out]
          n129 = Dequeue Element(queue=w487) -> (element=w486:string, error out=w477:errorcluster)  [unwired: 2 in, 2 out]
          n130 = call "PolInterpret.vi"("Format"=w484, "Time Bytes Before Output"=w479, "#Bytes"=w485, "Polhemus Output"=w486) -> ("Interpreted Values"=w480:sgl[], "Time"=w475:i32)
          "Interpreted Values" <- w480
          n131 = call "PolXYGraph.vi"("Interpreted Values"=w480, "x-indexes"=i32[] [1, 8], "y-indexes"=i32[] [2, 9] ("x-indexes")) -> ("XY Graph"=→"Hand Position Graph":cluster{sgl, sgl}[])  [unwired: 5 in]
          n132 = global read "GlobalVariables.vi" "Data Collect Stop"() -> (w478:bool)
          n133 = Divide(x=w475, y=1000.0) -> (x/y=→"Time":dbl)
          n134 = node-c288(w477) -> ()  [unwired: 1 out]
        }
        n135 = call "PolhemusDataCollect.vi"("Data Queue"=w467, "Timed Structure Name"="Polhemus", "VISA resource name"=w466, "Bytes to Read"=w464, "Relative Time"=w459, "error in (no error)"=w465, "Timed Loop Priority"=100, "Time Bytes Before Output"=w455, "Sync In? (F)"=w458) -> ("Queue Out"=w463:refnum<queue>, "VISA resource name out"=w454:refnum<visa-resource-name>, "error out"=w462:errorcluster)  [unwired: 3 in, 1 out]
        n136 = node-c288(w472) -> ()  [unwired: 1 out]
        n137 = Release Queue(queue=w463, error in (no error)=w462) -> ()  [unwired: 1 in, 3 out]
      }
    }
    n138 = case shown="True" w123 {
      selector: w123 -> [w235 w247]
      tunnel: w99 -> [_ w239]
      tunnel: w98 -> [_ w252]
      tunnel: w122 -> [_ w245]
      tunnel: w121 -> [_ w244]
      tunnel: [w235 w247] -> w115
      tunnel: w109 -> [_ w243]
      frame #0 {
      }
      frame #1 {
        n139 = Number To Decimal String(number=w252) -> (decimal integer string=w241:string)  [unwired: 1 in]
        n140 = Concatenate Strings("RH_Raw", w241) -> (w248:string)
        n141 = Concatenate Strings("RH_Deg", w241) -> (w249:string)
        n142 = Concatenate Strings("RH_Time", w241) -> (w240:string)
        n143 = Build Path(base path=w239, name or relative path=w249) -> (appended path=w236:path)
        n144 = Build Path(base path=w239, name or relative path=w240) -> (appended path=w237:path)
        n145 = Build Path(base path=w239, name or relative path=w248) -> (appended path=w238:path)
        n146 = call-poly <vilib>:"Write To Spreadsheet File.vi"("2D data"=w245, "file path (dialog if empty)"=w238) -> ()  [unwired: 6 in, 1 out]
        n147 = call-poly <vilib>:"Write To Spreadsheet File.vi"("2D data"=w244, "file path (dialog if empty)"=w236) -> ()  [unwired: 6 in, 1 out]
        n148 = call-poly <vilib>:"Write To Spreadsheet File.vi"("transpose? (no:F)"=TRUE, "1D data"=w243, "file path (dialog if empty)"=w237) -> ()  [unwired: 5 in, 1 out]
      }
    }
    n149 = case shown="True" w118 {
      selector: w118 -> [w217 w229]
      tunnel: w99 -> [_ w225]
      tunnel: w98 -> [_ w234]
      tunnel: w120 -> [_ w221]
      tunnel: w119 -> [_ w220]
      tunnel: [w217 w229] -> w114
      tunnel: w111 -> [_ w219]
      frame #0 {
      }
      frame #1 {
        n150 = Number To Decimal String(number=w234) -> (decimal integer string=w227:string)  [unwired: 1 in]
        n151 = Concatenate Strings("LH_Raw", w227) -> (w230:string)
        n152 = Concatenate Strings("LH_Time", w227) -> (w226:string)
        n153 = Concatenate Strings("LH_Deg", w227) -> (w231:string)
        n154 = Build Path(base path=w225, name or relative path=w231) -> (appended path=w223:path)
        n155 = Build Path(base path=w225, name or relative path=w226) -> (appended path=w222:path)
        n156 = Build Path(base path=w225, name or relative path=w230) -> (appended path=w224:path)
        n157 = call-poly <vilib>:"Write To Spreadsheet File.vi"("2D data"=w221, "file path (dialog if empty)"=w224) -> ()  [unwired: 6 in, 1 out]
        n158 = call-poly <vilib>:"Write To Spreadsheet File.vi"("2D data"=w220, "file path (dialog if empty)"=w223) -> ()  [unwired: 6 in, 1 out]
        n159 = call-poly <vilib>:"Write To Spreadsheet File.vi"("transpose? (no:F)"=TRUE, "1D data"=w219, "file path (dialog if empty)"=w222) -> ()  [unwired: 5 in, 1 out]
      }
    }
    n160 = case shown="True" w117 {
      selector: w117 -> [w253 w261]
      tunnel: w99 -> [_ w258]
      tunnel: w98 -> [_ w254]
      tunnel: w116 -> [_ w260]
      tunnel: [w253 w261] -> w113
      tunnel: w110 -> [_ w259]
      tunnel: w106 -> [_ w257]
      tunnel: w100 -> [_ w256]
      frame #0 {
      }
      frame #1 {
        # "PolTimes"
        # "Interp Vals"
        # "Time Marks"
        # "Titles"
        # "Trial#"
        # "Data Path"
        n161 = case shown="Default" w254 {
          selector: w254 -> [w262 _]
          tunnel: w260 -> [w271 w285]
          tunnel: w259 -> [w270 w286]
          tunnel: w258 -> [w265 w280]
          tunnel: w257 -> [w263 w281]
          tunnel: w256 -> [_ w287]
          tunnel: sgl[][] [] -> [_ w284]
          frame #0 {
            # "Normal Behavior"
            n162 = Number To Decimal String(number=w262) -> (decimal integer string=w273:string)  [unwired: 1 in]
            n163 = invoke on="Time" class="DigNum (strict)" method="Reinit To Default"() -> ()  [unwired: 3 in, 3 out]
            n164 = Concatenate Strings("Pol_Time" ("string"), w273) -> (w272:string)
            n165 = Concatenate Strings("Pol_Data" ("string"), w273) -> (w275:string)
            n166 = Build Path(base path=w265, name or relative path="Pol_Titles") -> (appended path=w264:path)
            n167 = Build Path(base path=w265, name or relative path=w272) -> (appended path=w268:path)
            n168 = Build Path(base path=w265, name or relative path=w275) -> (appended path=w267:path)
            n169 = call-poly <vilib>:"Write To Spreadsheet File.vi"("2D data"=w271, "file path (dialog if empty)"=w267) -> ()  [unwired: 6 in, 1 out]
            n170 = call-poly <vilib>:"Write To Spreadsheet File.vi"("transpose? (no:F)"=TRUE, "1D data"=w270, "file path (dialog if empty)"=w268) -> ()  [unwired: 5 in, 1 out]
            n171 = call-poly <vilib>:"Write To Spreadsheet File.vi"("1D data"=w263, "file path (dialog if empty)"=w264) -> ()  [unwired: 6 in, 1 out]
          }
          frame #1 {
            # "Records marks\nif Trial = 99"
            n172 = for {
              tunnel: w287 -> [w294] mode=indexing
              tunnel: w286 -> [w295]
              tunnel: w285 -> [w291]
              shift-right: [w289] -> w278
              shift-left: w284 -> [w288]
              # "First record after the mark"
              n173 = Subtract(x=w295, y=w294) -> (x-y=w293:u32[])
              n174 = Array Max & Min(array=w293) -> (min index (indices)=w292:i32)  [unwired: 3 out]
              n175 = Index Array(array=w291, index (row)=w292) -> (element=w290:sgl[])  [unwired: 1 in]
              n176 = Build Array (concatenate)(w288, w290) -> (w289:sgl[][])
            }
            n177 = Build Path(base path=w280, name or relative path="Pol_Titles") -> (appended path=w283:path)
            n178 = Build Path(base path=w280, name or relative path="Positions") -> (appended path=w277:path)
            n179 = call-poly <vilib>:"Write To Spreadsheet File.vi"("2D data"=w278, "file path (dialog if empty)"=w277) -> ()  [unwired: 6 in, 1 out]
            n180 = call-poly <vilib>:"Write To Spreadsheet File.vi"("1D data"=w281, "file path (dialog if empty)"=w283) -> ()  [unwired: 6 in, 1 out]
          }
        }
      }
    }
    n181 = case shown="True" w104 {
      tunnel: w100 -> [_ w166]
      tunnel: w99 -> [_ w165]
      tunnel: w98 -> [_ w163]
      tunnel: w97 -> [_ w164]
      frame #0 {
      }
      frame #1 {
        n182 = case shown="Default" w163 {
          selector: w163 -> [_ w169]
          tunnel: w166 -> [_ w178]
          tunnel: w165 -> [_ w172]
          tunnel: w164 -> [_ w173]
          frame #0 {
            # "Don't record the trial marks\nor trial number if doing\nposition marking."
          }
          frame #1 {
            n183 = Build Array(w169) -> (w168:i32[])
            n184 = Number To Decimal String(number=w169) -> (decimal integer string=w182:string)  [unwired: 1 in]
            n185 = Build Path(base path=w172, name or relative path="Trials") -> (appended path=w170:path)
            n186 = Concatenate Strings("TimeMarks" ("string"), w182) -> (w181:string)
            n187 = Build Path(base path=w172, name or relative path=w181) -> (appended path=w180:path)
            n188 = Build Path(base path=w172, name or relative path="TrialLengths") -> (appended path=w175:path)
            n189 = call-poly <vilib>:"Write To Spreadsheet File.vi"("append to file? (new file:F)"=TRUE, "1D data"=w168, "file path (dialog if empty)"=w170) -> ()  [unwired: 5 in, 1 out]
            n190 = Build Array(w173) -> (w176:u32[])
            n191 = call-poly <vilib>:"Write To Spreadsheet File.vi"("append to file? (new file:F)"=TRUE, "1D data"=w176, "file path (dialog if empty)"=w175) -> ()  [unwired: 5 in, 1 out]
            n192 = call-poly <vilib>:"Write To Spreadsheet File.vi"("transpose? (no:F)"=TRUE, "1D data"=w178, "file path (dialog if empty)"=w180) -> ()  [unwired: 5 in, 1 out]
          }
        }
      }
    }
    n193 = Compound Arithmetic op=OR(w115, w114, w113) -> (w112:bool)
    n194 = case shown="True" w112 {
      frame #0 {
      }
      frame #1 {
        # "Increment Trial\nonly if data colllection\noccured"
        n195 = local read "Trial #"() -> (w216:i32)
        n196 = Increment(x=w216) -> (x+1=w215:i32)
        n197 = local write "Trial #"(w215) -> ()
      }
    }
  }
  n198 = VISA Close(VISA resource name=w9) -> ()  [unwired: 1 in, 1 out]
  n199 = VISA Close(VISA resource name=w8) -> ()  [unwired: 1 in, 1 out]
  n200 = VISA Close(VISA resource name=w10) -> ()  [unwired: 1 in, 1 out]
  n201 = for {
    tunnel: w12 -> [w499] mode=indexing
    tunnel: [w497] -> _ mode=indexing
    # "Reenables the disabled controls"
    n202 = property class="Ctl"(reference=w499, "DisabledEnum"=T2."Enabled" ("Disabled")) -> (reference out=w497:refnum<vi>)  [unwired: 1 in, 1 out]
  }
